vi "Write command.vi"(8 "error in (no error)":errorcluster, 10 "command":refnum<k21>, 11 "Relay in":refnum<class "Relay.lvclass">) -> (0 "error out":errorcluster, 3 "Relay out":refnum<class "Relay.lvclass">)   [LabVIEW 2015]
uses:
  Relay.lvclass
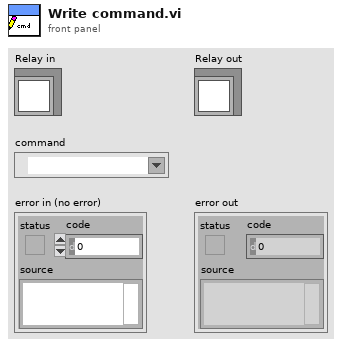
[diagram p1: front panel]
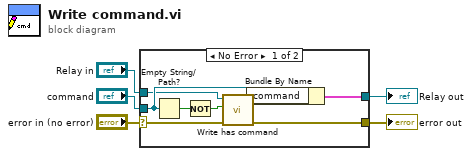
[diagram p0: block diagram]
diagram:
  n1 = case shown="No Error" "error in (no error)" {
    selector: "error in (no error)" -> [w7 w14]
    tunnel: [w6 w14] -> w4
    tunnel: [w13 w15] -> w2
    tunnel: "Relay in" -> [w9 w15]
    tunnel: "command" -> [w12 _]
    frame No Error {
      n2 = Empty String/Path?(string/path=w12) -> (empty?=w11:bool)
      n3 = Not(x=w11) -> (.not. x?=w10:bool)
      n4 = call "Write has command.vi"("error in (no error)"=w7, "has command"=w10, "Relay in"=w9) -> ("error out"=w6:errorcluster, "Relay out"=w8:refnum<class "Relay.lvclass">)  [unwired: 7 in]
      n5 = Bundle By Name(cluster=w8, "command"=w12) -> (w13:cluster{})
    }
    frame Error {
    }
  }
  "error out" <- w4
  "Relay out" <- w2
